vi "Variables Read for Position Control.vi"() -> (1 "Trajectory Trigger":i32, 5 "Start, End Point":bool[](array[boolean]))   [LabVIEW 2021]
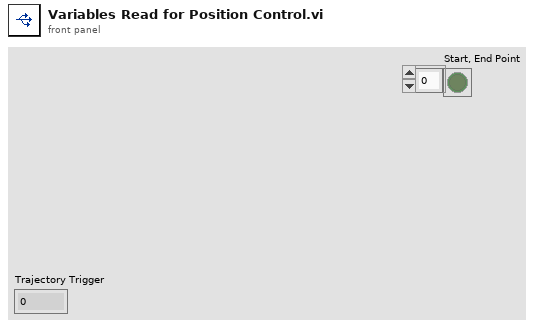
[diagram p1: front panel]
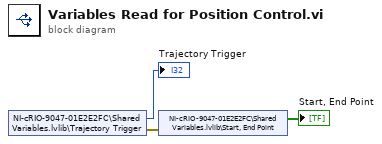
[diagram p0: block diagram]
diagram:
  n1 = shared-variable "NI-cRIO-9047-01E2E2FC\\Shared Variables.lvlib\\Trajectory Trigger"() -> (→"Trajectory Trigger":i32, error out=w1:errorcluster)  [unwired: 1 in]
  n2 = shared-variable "NI-cRIO-9047-01E2E2FC\\Shared Variables.lvlib\\Start, End Point"(error in=w1) -> (→"Start, End Point":bool[])  [unwired: 1 out]
